vi "RunTestSuite--function.vi"(4 "timeout (s) (2000)":i32, 6 "Verbose (F)":bool, 8 "error in":errorcluster, 9 "Interactive (F)":bool, 10 "Report Path":path, 11 "Test Suite (.vi)":path) -> (0 "error out":errorcluster, 1 "test error":errorcluster, 2 "Report Path":path)   [LabVIEW 2020, in "CICD.lvlib"]
doc: "Run Tests using Caraya Unit Test Framework."
uses:
  CICD.lvlib
  Test VI Type Specifier.vi
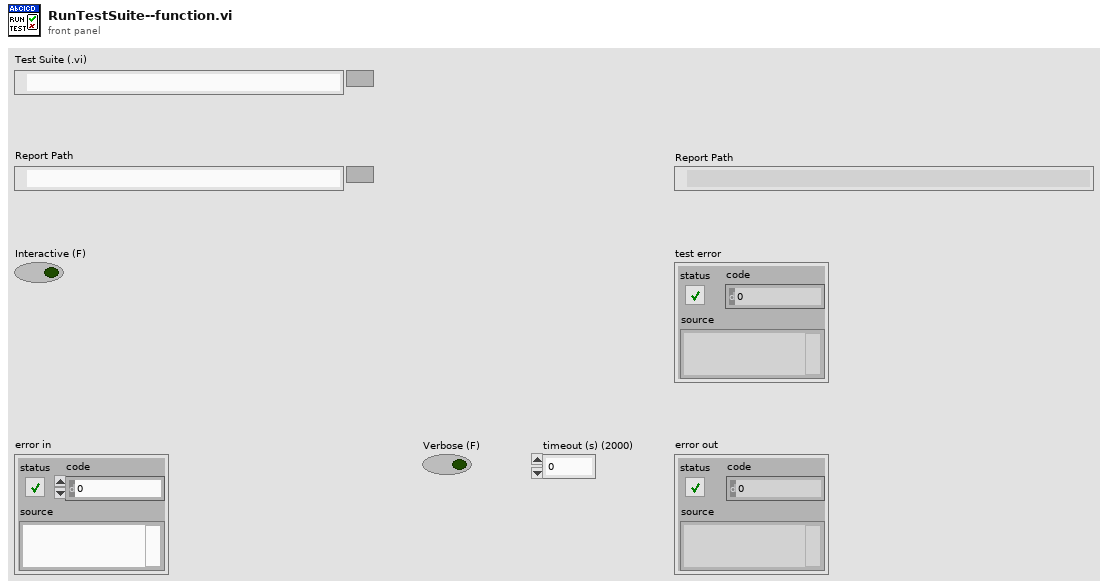
[diagram p1: front panel]
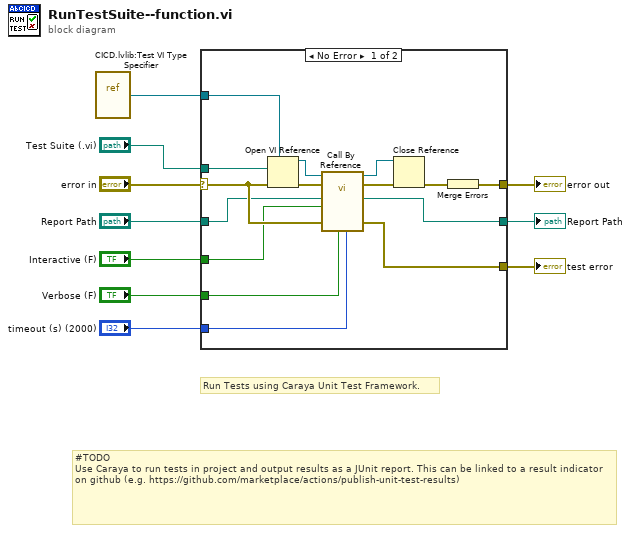
[diagram p0: block diagram]
diagram:
  # "#TODO\nUse Caraya to run tests in project and output results as a JUnit report. This can be linked to a result indicator on github (e.g. https://github.com/marketplace/actions/publish-unit-test-results)"
  # "Run Tests using Caraya Unit Test Framework."
  n1 = vi-ref "CICD.lvlib:Test VI Type Specifier.vi"() -> (w3:refnum<vi>)
  n2 = case shown="No Error" "error in" {
    selector: "error in" -> [w21 w27]
    tunnel: [w22 w27] -> w10
    tunnel: w3 -> [w19 _]
    tunnel: "Report Path" -> [w17 w26]
    tunnel: "Test Suite (.vi)" -> [w16 _]
    tunnel: [w14 w26] -> w5
    tunnel: "Interactive (F)" -> [w13 _]
    tunnel: [w20 _] -> w8
    tunnel: "Verbose (F)" -> [w12 _]
    tunnel: "timeout (s) (2000)" -> [w11 _]
    frame No Error {
      n3 = Open VI Reference(type specifier VI Refnum (for type only)=w19, vi path=w16, error in (no error)=w21) -> (vi reference=w18:refnum<vi>, error out=w24:errorcluster)  [unwired: 3 in]
      n4 = call-by-ref "?"(reference=w18, error in=w24, "timeout (s) (2000)"=w11, "Verbose (F)"=w12, "error in"=w21, "Interactive (F)"=w13, "Report Path"=w17) -> (reference out=w15:refnum<vi>, error out=w25:errorcluster, 0:"error out"=w20:errorcluster, "Report Path"=w14:path)  [unwired: 5 in]
      n5 = Close Reference(reference=w15, error in (no error)=w25) -> (error out=w23:errorcluster)
      n6 = Merge Errors(w23) -> (w22:errorcluster)
    }
    frame Error {
    }
  }
  "error out" <- w10
  "Report Path" <- w5
  "test error" <- w8
